vi "Stitching-Generate canvas template.vi"(6 "Experiment folder names column to use":i32, 8 "error in (no error)":errorcluster, 9 "Selected rows":i32[](array[numeric]), 10 "Item Names":string[][](array[string]), 11 "Base directory containing all dataset folders":path) -> (0 "error out":errorcluster, 1 "Min":cluster{"X min (um) ":dbl, "Y min (um)":dbl}, 2 "Single image size (pixels)":i32, 3 "Canvas":T2, 4 "Cancelled?":bool, 5 "Stitched image setup":T1)   [LabVIEW 2013]
uses:
  <vilib>/vision/Image Controls.llb/IMAQ Image.ctl
  Coordinates list window/Globals/Coord window-Globals.vi
panel:
  out "Canvas Y size (um)":dbl
  out "Canvas X size (um)":dbl
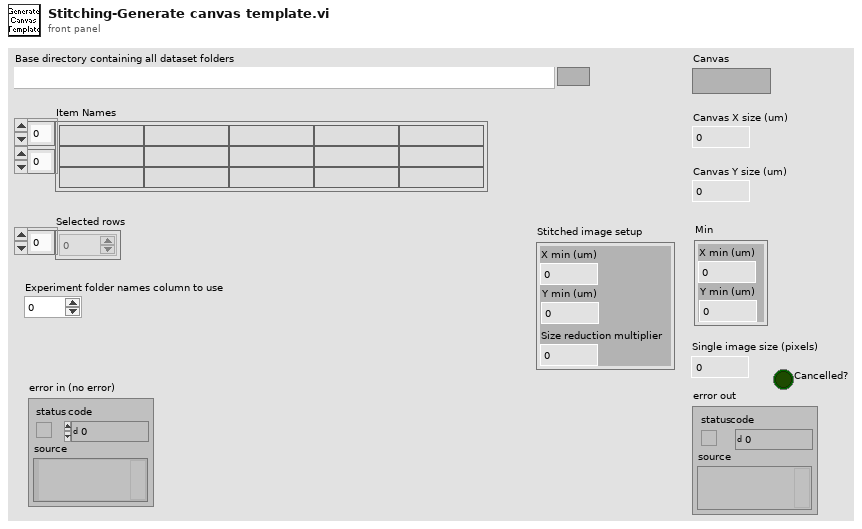
[diagram p1: front panel]
types:
  T1 = cluster{"X min (um) ":i32, "Y min (um)":i32, "Size reduction multiplier":dbl}
  T2 = typedef "IMAQ Image.ctl" = refnum<image>
  T3 = typedef "Image Type" = u32
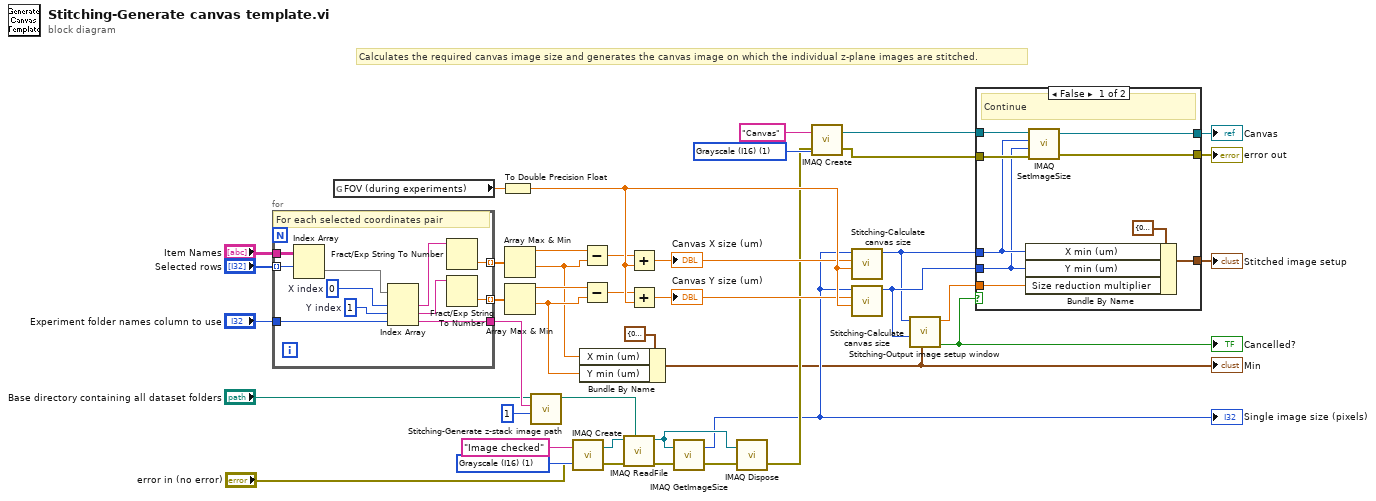
[diagram p0: block diagram]
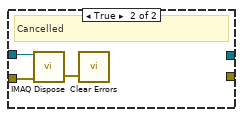
[diagram p2: hidden frame]
diagram:
  w35 = T3 1 items=["Grayscale (U8)", "Grayscale (I16)", "Grayscale (SGL)", "Complex (CSG)", "RGB (U32)", "HSL (U32)", "RGB (U64)", "Grayscale (U16)"] ("Image Type")
  w13 = T3 1 items=["Grayscale (U8)", "Grayscale (I16)", "Grayscale (SGL)", "Complex (CSG)", "RGB (U32)", "HSL (U32)", "RGB (U64)", "Grayscale (U16)"] ("Image Type")
  # "Calculates the required canvas image size and generates the canvas image on which the individual z-plane images are stitched."
  n1 = for {
    tunnel: "Selected rows" -> [w52] mode=indexing
    tunnel: "Item Names" -> [w53]
    tunnel: [w46] -> w30 mode=indexing
    tunnel: [w45] -> w25 mode=indexing
    tunnel: [w44] -> w33
    tunnel: "Experiment folder names column to use" -> [w43]
    w49 = 1  # Y index
    w50 = 0  # X index
    # "For each selected coordinates pair"
    n2 = Index Array(array=w53, index (row)=w52) -> (element=w51:string[])  [unwired: 1 in]
    n3 = Index Array(array=w51, index #1=w50, index #2=w49, index #3=w43) -> (element #1=w48:string, element #2=w47:string, element #3=w44:string)
    n4 = Fract/Exp String To Number(string=w48) -> (number=w46:dbl)  [unwired: 3 in, 1 out]
    n5 = Fract/Exp String To Number(string=w47) -> (number=w45:dbl)  [unwired: 3 in, 1 out]
  }
  n6 = global read "Coord window-Globals.vi" "FOV (during experiments)"() -> (w23:sgl)
  n7 = To Double Precision Float(number=w23) -> (double precision float=w42:dbl)
  n8 = Array Max & Min(array=w30) -> (max value=w29:dbl, min value=w17:dbl)  [unwired: 2 out]
  n9 = Array Max & Min(array=w25) -> (max value=w26:dbl, min value=w18:dbl)  [unwired: 2 out]
  n10 = call "Stitching-Generate z-stack image path.vi"("File increment number / Z-plane number"=1 ("Numeric"), "Experiment folder name"=w33, "Base directory"="Base directory containing all dataset folders") -> ("appended path"=w38:path)  [unwired: 8 in]
  n11 = call "IMAQ Create"("Image Name"="Image checked", "Image Type"=w35, "error in (no error)"="error in (no error)") -> ("New Image"=w37:T2, "error out"=w16:errorcluster)  [unwired: 2 in]
  n12 = Bundle By Name(cluster=cluster{"X min (um) ":dbl, "Y min (um)":dbl} {"X min (um) "=0.0, "Y min (um)"=0.0} ("Min"), "X min (um)"=w17, "Y min (um)"=w18) -> (w4:cluster{"X min (um) ":dbl, "Y min (um)":dbl})
  "Min" <- w4
  n13 = Subtract(x=w29, y=w17) -> (x-y=w28:dbl)
  n14 = Subtract(x=w26, y=w18) -> (x-y=w27:dbl)
  n15 = call "IMAQ ReadFile"("File Path"=w38, "error in (no error)"=w16, "Image"=w37) -> ("error out"=w11:errorcluster, "Image Out"=w8:T2)  [unwired: 4 in, 3 out]
  n16 = Add(x=w28, y=w42) -> (x+y=w40:dbl)
  "Canvas X size (um)" <- w40
  n17 = Add(x=w27, y=w42) -> (x+y=w41:dbl)
  "Canvas Y size (um)" <- w41
  n18 = call "IMAQ GetImageSize"("Image"=w8, "error in (no error)"=w11) -> ("Y Resolution"=w7:i32, "error out"=w10:errorcluster)  [unwired: 3 out]
  "Single image size (pixels)" <- w7
  n19 = call "IMAQ Dispose"("Image"=w8, "error in (no error)"=w10) -> ("error out"=w9:errorcluster)  [unwired: 4 in]
  n20 = call "IMAQ Create"("Image Name"="Canvas", "Image Type"=w13, "error in (no error)"=w9) -> ("New Image"=w39:T2, "error out"=w15:errorcluster)  [unwired: 2 in]
  n21 = call "Stitching-Calculate canvas size.vi"("FOV (um)"=w42, "Canvas size (um)"=w40, "Single image size (pixels)"=w7) -> ("Canvas size (pixels)"=w2:i32)  [unwired: 8 in]
  n22 = call "Stitching-Calculate canvas size.vi"("FOV (um)"=w42, "Canvas size (um)"=w41, "Single image size (pixels)"=w7) -> ("Canvas size (pixels)"=w3:i32)  [unwired: 8 in]
  n23 = call "Stitching-Output image setup window.vi"("Min"=w4, "Canvas Y size in"=w3, "Canvas X size in"=w2) -> ("Cancelled?"=w5:bool, "Size reduction multiplier"=w1:dbl)  [unwired: 7 in]
  "Cancelled?" <- w5
  n24 = case shown="False" w5 {
    tunnel: w39 -> [w62 w65]
    tunnel: [w61 _] -> w21
    tunnel: w15 -> [w60 w64]
    tunnel: [w59 _] -> w14
    tunnel: [w57 _] -> w6
    tunnel: w2 -> [w56 _]
    tunnel: w3 -> [w55 _]
    tunnel: w1 -> [w54 _]
    frame False {
      # "Continue"
      n25 = Bundle By Name(cluster=T1 {"X min (um) "=0, "Y min (um)"=0, "Size reduction multiplier"=0.0} ("Min"), "X min (um)"=w56, "Y min (um)"=w55, "Size reduction multiplier"=w54) -> (w57:T1)
      n26 = call "IMAQ SetImageSize"("error in (no error)"=w60, "Y Resolution"=w55, "X Resolution"=w56, "Image"=w62) -> ("error out"=w59:errorcluster, "Image Out"=w61:T2)  [unwired: 1 out]
    }
    frame True {
      # "Cancelled"
      n27 = call "IMAQ Dispose"("Image"=w65, "error in (no error)"=w64) -> ("error out"=w63:errorcluster)  [unwired: 4 in]
      n28 = call <vilib>:"Clear Errors.vi"("error in (no error)"=w63) -> ()  [unwired: 6 in, 1 out]
    }
  }
  "Canvas" <- w21
  "error out" <- w14
  "Stitched image setup" <- w6
